vi "dlw_TCP Read.vi"(6 "Worker Alias":string="TCP Read", 7 "Caller in":refnum<class "Worker.lvclass">, 8 "error in":errorcluster, 9 "Initialization Data":T1, 11 "TCP Read in":refnum<class "TCP Read.lvclass">) -> (0 "error out":errorcluster, 3 "TCP Read out":refnum<class "TCP Read.lvclass">, 5 "dup Caller out":refnum<class "Worker.lvclass">)   [LabVIEW 2017, in "_TCP Server.lvlib" / "TCP Read.lvclass"]
doc: "This VI dynamically loads the Worker that owns this VI as a subWorker into <b>Caller</b>, and returns the Worker's object containing the Worker's Public Accessible data. Initialization data that is to be received by this Worker's <Initialize> MHL case can be wired to <b>Initialization Data</b>. The dynamically loaded Worker requires an alias ( <b>Worker Alias</b> ) which must be unique to the Worker it is called from. If a currently loaded subWorker exists with the same Alias, an error will be returned.\n\n<b>Note:</b> This VI can only be called from <b>within</b> another Worker. To call this Worker from an external LabVIEW application, load this Worker with an Asynchronous Launcher VI.\n---"
uses:
  TCP Read.lvclass
  C:/SC/Source Code/VIPM/LabVIEW 20xx/vi.lib/addons/_Workers/Library/Classes/Worker/Worker.lvclass
  <vilib>/addons/_Workers/Library/Classes/Worker/Worker.lvclass
  Initialization Data.ctl
  <vilib>/addons/_Workers/Library/Classes/Message Queue/Message Queue.lvclass
  Response Cases.ctl
  <vilib>/addons/_Workers/Library/Case Label.ctl
  <vilib>/addons/_Workers/Library/Workers.lvlib
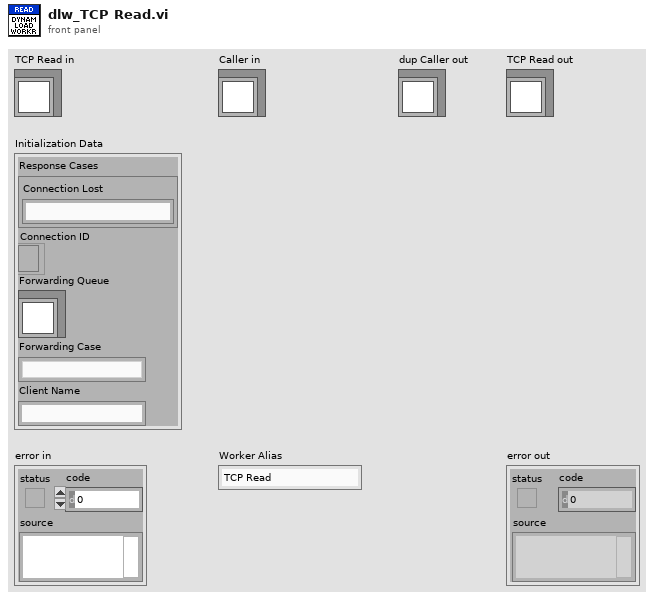
[diagram p1: front panel]
types:
  T1 = typedef "_TCP Server.lvlib/TCP Read.lvclass/Initialization Data.ctl" = cluster{"Response Cases":T2, "Connection ID":refnum<k5>, "Forwarding Queue":refnum<class "Message Queue.lvclass">, "Forwarding Case":T3, "Client Name":string}
  T2 = typedef "_TCP Server.lvlib/TCP Read.lvclass/Response Cases.ctl" = cluster{"Connection Lost":T3}
  T3 = typedef "Workers.lvlib/Case Label.ctl" = string
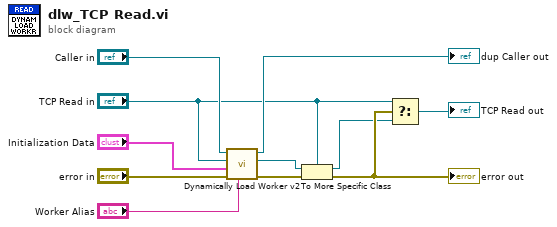
[diagram p0: block diagram]
diagram:
  n1 = call <vilib>:"Dynamically Load Worker v2.vi"("Worker Alias"="Worker Alias", "error in"="error in", "Initialization Data"="Initialization Data", "Worker to Dynamically Load"="TCP Read in", "Worker"="Caller in") -> ("error out"=w10:errorcluster, "Dynamically Loaded Worker out"=w5:refnum<class "Worker.lvclass">, "dup Worker out"=→"dup Caller out":refnum<class "Worker.lvclass">)  [unwired: 4 in]
  n2 = To More Specific Class(target class="TCP Read in", reference=w5, error in=w10) -> (specific class reference=w2:refnum<class "TCP Read.lvclass">, error out=w4:errorcluster)
  "error out" <- w4
  n3 = Select(t="TCP Read in", s=w4, f=w2) -> (s? t:f=→"TCP Read out":refnum<class "TCP Read.lvclass">)
